vi "Conversão_Valores_CLP_Instrumentos.vi"(1 "String":string, 2 "MIN":dbl, 3 "MAX":dbl, 4 "CLP":dbl) -> (0 "S":dbl)   [LabVIEW 2019]
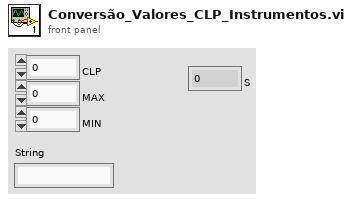
[diagram p1: front panel]
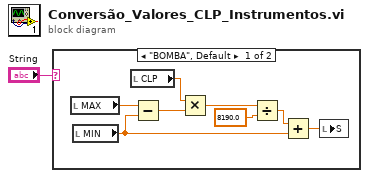
[diagram p0: block diagram]
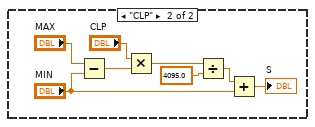
[diagram p2: hidden frame]
diagram:
  n1 = case shown="\"BOMBA\", Default" "String" {
    frame "BOMBA", Default {
      n2 = local read "MAX"() -> (w3:dbl)
      n3 = local read "MIN"() -> (w2:dbl)
      n4 = local read "CLP"() -> (w4:dbl)
      n5 = Subtract(x=w3, y=w2) -> (x-y=w9:dbl)
      n6 = Multiply(x=w4, y=w9) -> (x*y=w8:dbl)
      n7 = Divide(x=w8, y=8190.0) -> (x/y=w7:dbl)
      n8 = Add(x=w7, y=w2) -> (x+y=w5:dbl)
      n9 = local write "S"(w5) -> ()
    }
    frame "CLP" {
      n10 = Subtract(x="MAX", y="MIN") -> (x-y=w16:dbl)
      n11 = Multiply(x="CLP", y=w16) -> (x*y=w14:dbl)
      n12 = Divide(x=w14, y=4095.0) -> (x/y=w12:dbl)
      n13 = Add(x=w12, y="MIN") -> (x+y=→"S":dbl)
    }
  }
